vi "Bearing_Clust_Test_Panel.vi"(8 "error in (no error)":errorcluster) -> (0 "error out":errorcluster)   [LabVIEW 2019, in "MHL.lvlib"]
uses:
  MHL.lvlib
  typedef/Alarm_Panel.ctl
  Alarm_Panel/Channel_Temperature_Threshold.ctl
  typedef/MHL_Data.ctl
panel:
  in  "Alarm Panel":T1
  out "Bearing Temp Data":T3 {"[0]" format="%#_g °C"; "[1]" format="%#_g °C"; "[6]" format="%#_g °C"; "[7]" format="%#_g °C"; "[10]" format="%#_g °C"; "[11]" format="%#_g °C"; "[2]" format="%#_g °C"; "[3]" format="%#_g °C"; "[4]" format="%#_g °C"; "[5]" format="%#_g °C"; "[8]" format="%#_g °C"; "[9]" format="%#_g °C"; "[12]" format="%#_g °C"; "[13]" format="%#_g °C"; "[14]" format="%#_g °C"; "[15]" format="%#_g °C"}
  # "Min"
  # "Max"
  # "Alarm"
  # "Min"
  # "Max"
  # "Alarm"
  # "Min"
  # "Max"
  # "Alarm"
  # "Min"
  # "Max"
  # "Alarm"
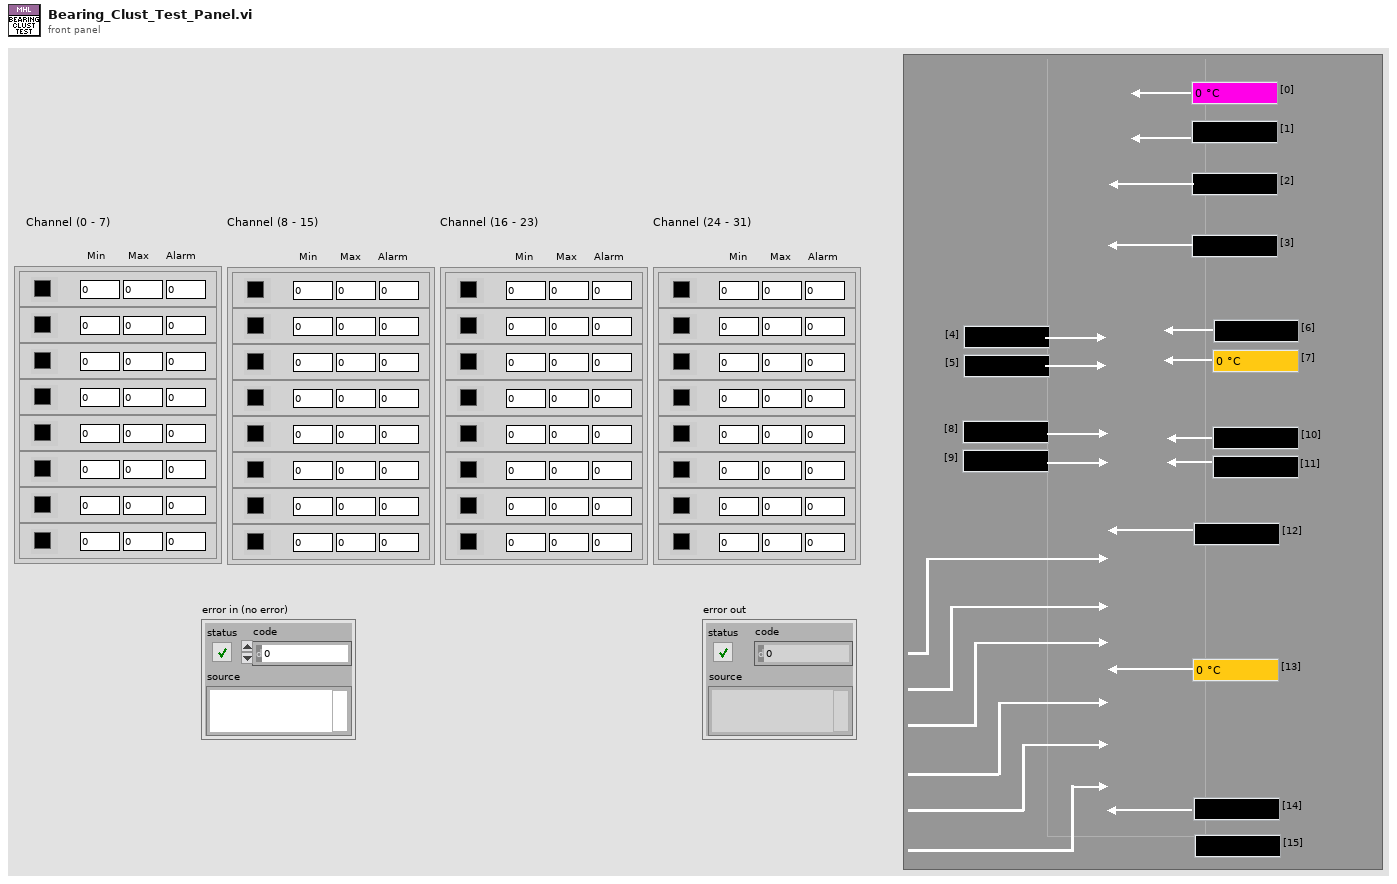
[diagram p1: front panel]
types:
  T1 = typedef "Alarm_Panel.ctl" = cluster{"Channel (0 - 7)":cluster{"Channel Temperature Thresholds":T2, "Channel Temperature Thresholds 2":T2, "Channel Temperature Thresholds 3":T2, "Channel Temperature Thresholds 4":T2, "Channel Temperature Thresholds 5":T2, "Channel Temperature Thresholds 6":T2, "Channel Temperature Thresholds 7":T2, "Channel Temperature Thresholds 8":T2}, "Channel (8 - 15)":cluster{"Channel Temperature Thresholds":T2, "Channel Temperature Thresholds 2":T2, "Channel Temperature Thresholds 3":T2, "Channel Temperature Thresholds 4":T2, "Channel Temperature Thresholds 5":T2, "Channel Temperature Thresholds 6":T2, "Channel Temperature Thresholds 7":T2, "Channel Temperature Thresholds 8":T2}, "Channel (16 - 23)":cluster{"Channel Temperature Thresholds":T2, "Channel Temperature Thresholds 2":T2, "Channel Temperature Thresholds 3":T2, "Channel Temperature Thresholds 4":T2, "Channel Temperature Thresholds 5":T2, "Channel Temperature Thresholds 6":T2, "Channel Temperature Thresholds 7":T2, "Channel Temperature Thresholds 8":T2}, "Channel (24 - 31)":cluster{"Channel Temperature Thresholds":T2, "Channel Temperature Thresholds 2":T2, "Channel Temperature Thresholds 3":T2, "Channel Temperature Thresholds 4":T2, "Channel Temperature Thresholds 5":T2, "Channel Temperature Thresholds 6":T2, "Channel Temperature Thresholds 7":T2, "Channel Temperature Thresholds 8":T2}}
  T2 = typedef "Channel_Temperature_Threshold.ctl" = cluster{"Min":i32, "Max":i32, "Alarm":i32, "Status":u32}
  T3 = cluster{"[0]":sgl, "[1]":sgl, "[2]":sgl, "[3]":sgl, "[4]":sgl, "[5]":sgl, "[6]":sgl, "[7]":sgl, "[8]":sgl, "[9]":sgl, "[10]":sgl, "[11]":sgl, "[12]":sgl, "[13]":sgl, "[14]":sgl, "[15]":sgl}
  T4 = typedef "MHL.lvlib/MHL_Data.ctl" = cluster{"Ctrl_Refs":cluster{"Quit":refnum<vi>, "Motor_Switch":refnum<vi>, "Status":refnum<vi>, "Alarm_Panel":refnum<vi>, "Bearing Temp Chart":refnum<vi>, "Motor Temp Chart":refnum<vi>, "TabCtl":refnum<vi>, "Bearing Temp Clust":refnum<vi>}, "Main_Ref":refnum<vi>}
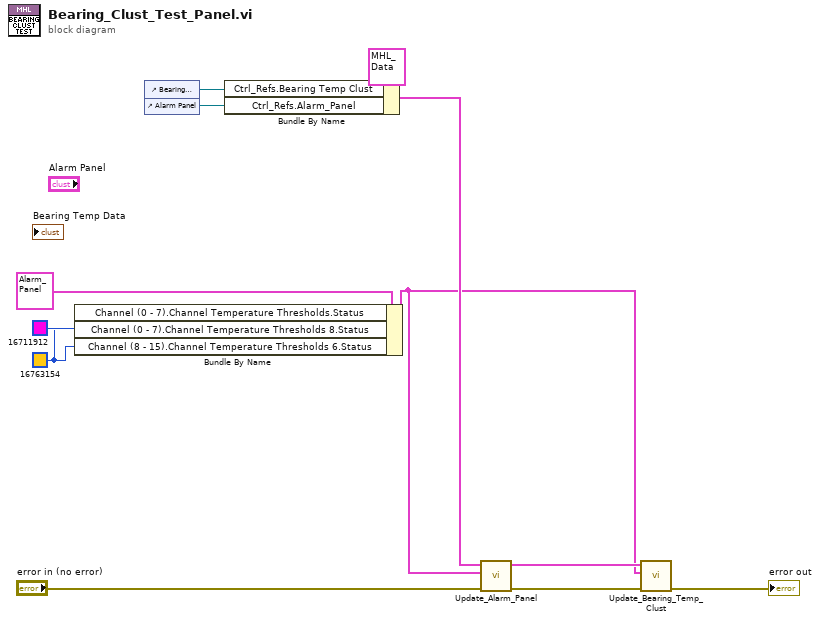
[diagram p0: block diagram]
diagram:
  w1 = u32 16763154
  n1 = Bundle By Name(cluster=T1 {"Channel (0 - 7)"={"Channel Temperature Thresholds"={"Min"=0, "Max"=0, "Alarm"=0, "Status"=0}, "Channel Temperature Thresholds 2"={"Min"=0, "Max"=0, "Alarm"=0, "Status"=0}, "Channel Temperature Thresholds 3"={"Min"=0, "Max"=0, "Alarm"=0, "Status"=0}, "Channel Temperature Thresholds 4"={"Min"=0, "Max"=0, "Alarm"=0, "Status"=0}, "Channel Temperature Thresholds 5"={"Min"=0, "Max"=0, "Alarm"=0, "Status"=0}, "Channel Temperature Thresholds 6"={"Min"=0, "Max"=0, "Alarm"=0, "Status"=0}, "Channel Temperature Thresholds 7"={"Min"=0, "Max"=0, "Alarm"=0, "Status"=0}, "Channel Temperature Thresholds 8"={"Min"=0, "Max"=0, "Alarm"=0, "Status"=0}}, "Channel (8 - 15)"={"Channel Temperature Thresholds"={"Min"=0, "Max"=0, "Alarm"=0, "Status"=0}, "Channel Temperature Thresholds 2"={"Min"=0, "Max"=0, "Alarm"=0, "Status"=0}, "Channel Temperature Thresholds 3"={"Min"=0, "Max"=0, "Alarm"=0, "Status"=0}, "Channel Temperature Thresholds 4"={"Min"=0, "Max"=0, "Alarm"=0, "Status"=0}, "Channel Temperature Thresholds 5"={"Min"=0, "Max"=0, "Alarm"=0, "Status"=0}, "Channel Temperature Thresholds 6"={"Min"=0, "Max"=0, "Alarm"=0, "Status"=0}, "Channel Temperature Thresholds 7"={"Min"=0, "Max"=0, "Alarm"=0, "Status"=0}, "Channel Temperature Thresholds 8"={"Min"=0, "Max"=0, "Alarm"=0, "Status"=0}}, "Channel (16 - 23)"={"Channel Temperature Thresholds"={"Min"=0, "Max"=0, "Alarm"=0, "Status"=0}, "Channel Temperature Thresholds 2"={"Min"=0, "Max"=0, "Alarm"=0, "Status"=0}, "Channel Temperature Thresholds 3"={"Min"=0, "Max"=0, "Alarm"=0, "Status"=0}, "Channel Temperature Thresholds 4"={"Min"=0, "Max"=0, "Alarm"=0, "Status"=0}, "Channel Temperature Thresholds 5"={"Min"=0, "Max"=0, "Alarm"=0, "Status"=0}, "Channel Temperature Thresholds 6"={"Min"=0, "Max"=0, "Alarm"=0, "Status"=0}, "Channel Temperature Thresholds 7"={"Min"=0, "Max"=0, "Alarm"=0, "Status"=0}, "Channel Temperature Thresholds 8"={"Min"=0, "Max"=0, "Alarm"=0, "Status"=0}}, "Channel (24 - 31)"={"Channel Temperature Thresholds"={"Min"=0, "Max"=0, "Alarm"=0, "Status"=0}, "Channel Temperature Thresholds 2"={"Min"=0, "Max"=0, "Alarm"=0, "Status"=0}, "Channel Temperature Thresholds 3"={"Min"=0, "Max"=0, "Alarm"=0, "Status"=0}, "Channel Temperature Thresholds 4"={"Min"=0, "Max"=0, "Alarm"=0, "Status"=0}, "Channel Temperature Thresholds 5"={"Min"=0, "Max"=0, "Alarm"=0, "Status"=0}, "Channel Temperature Thresholds 6"={"Min"=0, "Max"=0, "Alarm"=0, "Status"=0}, "Channel Temperature Thresholds 7"={"Min"=0, "Max"=0, "Alarm"=0, "Status"=0}, "Channel Temperature Thresholds 8"={"Min"=0, "Max"=0, "Alarm"=0, "Status"=0}}} ("Alarm Panel"), "Channel (0 - 7).Channel Temperature Thresholds.Status"=u32 16711912, "Channel (0 - 7).Channel Temperature Thresholds 8.Status"=w1, "Channel (8 - 15).Channel Temperature Thresholds 6.Status"=w1) -> (w3:T1)
  n2 = control-ref of="Bearing Temp Data"() -> (w7:refnum<vi>)
  n3 = control-ref of="Alarm Panel"() -> (w5:refnum<vi>)
  n4 = Bundle By Name(cluster=T4 {"Ctrl_Refs"={"Quit"=refnum, "Motor_Switch"=refnum, "Status"=refnum, "Alarm_Panel"=refnum, "Bearing Temp Chart"=refnum, "Motor Temp Chart"=refnum, "TabCtl"=refnum, "Bearing Temp Clust"=refnum}, "Main_Ref"=refnum} ("MHL_Data In"), "Ctrl_Refs.Bearing Temp Clust"=w7, "Ctrl_Refs.Alarm_Panel"=w5) -> (w8:T4)
  n5 = call "Update_Alarm_Panel.vi"("error in (no error)"="error in (no error)", "Data"=w3, "MHL_Data In"=w8) -> ("error out"=w11:errorcluster, "MHL_Data Out"=w6:T4)  [unwired: 7 in]
  n6 = call "Update_Bearing_Temp_Clust.vi"("error in (no error)"=w11, "Data In"=w3, "MHL_Data In"=w6) -> ("error out"=→"error out":errorcluster)  [unwired: 7 in, 1 out]
